vi "Begin.vi"(8 "error in":errorcluster) -> (0 "error out":errorcluster)   [LabVIEW 2020]
doc: "Called before other user functions, this VI is expected to open initial I/O refnums, load in file data, and do all program initialization. Notice that the <B>error out</B> terminal is simply used for data flow. Wiring it to other structures or subVIs ensures that this VI runs first."
uses:
  <vilib>/Rock Robotics/WPI/DriverStation/WPI_DriverStationRobotMode2.ctl
  <vilib>/Rock Robotics/WPI/Joystick/WPI_JoystickDeviceEnum.ctl
  <vilib>/Rock Robotics/WPI/SafetyOutput/WPI_SafetyOutputConfigMenu.ctl
  Robot Global Data.vi
  <vilib>/Rock Robotics/Network Tables/NT Write String Array.vi
  <vilib>/Rock Robotics/WPI/RobotDrive/WPI_RobotDriveOpen2MotorWithExistingMotors.vi
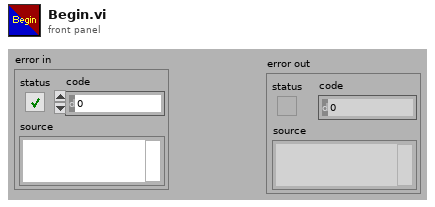
[diagram p1: front panel]
types:
  T1 = typedef "WPI_SafetyOutputConfigMenu.ctl" = enum16{"Enable", "Disable"}
  T2 = typedef "WPI_JoystickDeviceEnum.ctl" = enum16{"USB 0", "USB 1", "USB 2", "USB 3", "USB 4", "USB 5"}
  T3 = typedef "WPI_DriverStationRobotMode2.ctl" = enum16{"Autonomous Disabled", "Autonomous Enabled", "Teleop Disabled", "Teleop Enabled", "Disconnected", "Finish", "Test Disabled", "Test Enabled", "Emergency Stopped"}
  T4 = typedef "WPI_MotorControlDeviceRef.ctl" = cluster{"DeviceStatus":errorcluster, "Type":T5, "PWM":cluster{"PWM Channel":T6, "DeadBand":T7}, "CAN":cluster{"Device Number":u8, "SetOutput VI Ref":variant, "GetOutput VI Ref":variant, "Enable VI Ref":variant, "Disable VI Ref":variant, "Data":variant}, "Invert":bool, "DIO PWM":cluster{"PWM \"Enable\" Channel":T6, "DIOChannel":T8, "PWM Rate":dbl}}
  T5 = typedef "WPI_MotorControlType.ctl" = enum16{"PWM", "CAN", "DIO PWM"}
  T6 = typedef "FPGA_DIOPWMChannel.ctl" = enum8{"PWM 0", "PWM 1", "PWM 2", "PWM 3", "PWM 4", "PWM 5", "PWM 6", "PWM 7", "PWM 8", "PWM 9", "PWM MXP 0", "PWM MXP 1", "PWM MXP 2", "PWM MXP 3", "PWM MXP 4", "PWM MXP 5", "PWM MXP 6", "PWM MXP 7", "PWM MXP 8", "PWM MXP 9", "Invalid"}
  T7 = typedef "WPI_PWMDeadband.ctl" = cluster{"Name":string, "maxPositivePwm":i32, "minPositivePwm":i32, "centerPwm":i32, "maxNegativePwm":i32, "minNegativePwm":i32, "angularRange":u16}
  T8 = typedef "FPGA_DIOChannel.ctl" = enum8{"DIO 0", "DIO 1", "DIO 2", "DIO 3", "DIO 4", "DIO 5", "DIO 6", "DIO 7", "DIO 8", "DIO 9", "DIO MXP 0", "DIO MXP 1", "DIO MXP 2", "DIO MXP 3", "DIO MXP 4", "DIO MXP 5", "DIO MXP 6", "DIO MXP 7", "DIO MXP 8", "DIO MXP 9", "DIO MXP 10", "DIO MXP 11", "DIO MXP 12", "DIO MXP 13", "DIO MXP 14", "DIO MXP 15", "SPI Port CS1", "SPI Port CS2", "SPI Port CS3", "SPI Port MISO", "SPI Port MOSI", "Invalid"}
  T9 = typedef "WPI_JoystickDevRef.ctl" = cluster{"Device":T2}
  T10 = typedef "WPI_RobotDriveDevRef.ctl" = cluster{"DevStatus":errorcluster, "Motors[]":T4[], "Square Inputs":bool, "Max Output":dbl}
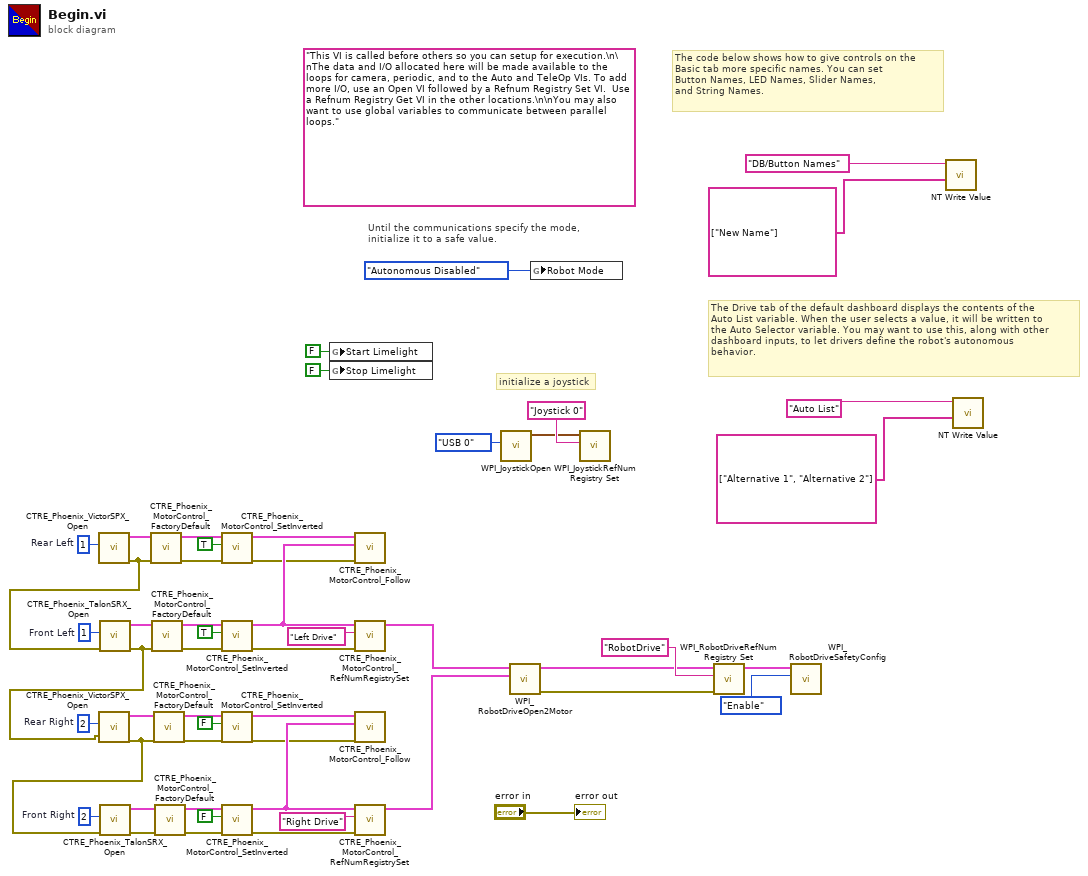
[diagram p0: block diagram]
diagram:
  w35 = u8 2  # Front Right
  w34 = u8 2  # Rear Right
  w33 = u8 1  # Front Left
  w32 = u8 1  # Rear Left
  (unwired) "This VI is called before others so you can setup for execution.\n\nThe data and I/O allocated here will be made available to the loops for camera, periodic, and to the Auto and TeleOp VIs. To add more I/O, use an Open VI followed by a Refnum Registry Set VI.  Use a Refnum Registry Get VI in the other locations.\n\nYou may also want to use global variables to communicate between parallel loops."
  # "The Drive tab of the default dashboard displays the contents of the\nAuto List variable. When the user selects a value, it will be written to\nthe Auto Selector variable. You may want to use this, along with other\ndashboard inputs, to let drivers define the robot's autonomous\nbehavior."
  # "The code below shows how to give controls on the\nBasic tab more specific names. You can set\nButton Names, LED Names, Slider Names,\nand String Names."
  # "initialize a joystick"
  # "Until the communications specify the mode,\ninitialize it to a safe value."
  n1 = call <vilib>:"CTRE_Phoenix_VictorSPX_Open.vi"("Device Number"=w32) -> ("error out"=w38:errorcluster, "PhoenixMotorControlDevRef"=w5:T4)  [unwired: 9 in]
  n2 = call <vilib>:"CTRE_Phoenix_TalonSRX_Open.vi"("error in"=w38, "Device Number"=w33) -> ("error out"=w39:errorcluster, "PhoenixMotorControlDevRef"=w11:T4)  [unwired: 8 in]
  n3 = call <vilib>:"CTRE_Phoenix_VictorSPX_Open.vi"("error in"=w39, "Device Number"=w34) -> ("error out"=w40:errorcluster, "PhoenixMotorControlDevRef"=w6:T4)  [unwired: 8 in]
  n4 = call <vilib>:"CTRE_Phoenix_TalonSRX_Open.vi"("error in"=w40, "Device Number"=w35) -> ("error out"=w12:errorcluster, "PhoenixMotorControlDevRef"=w13:T4)  [unwired: 8 in]
  n5 = call <vilib>:"CTRE_Phoenix_MotorControl_FactoryDefault.vi"("error in"=w38, "PhoenixMotorControlDevRef"=w5) -> ("error out"=w9:errorcluster, "PhoenixMotorControlDevRef"=w10:T4)  [unwired: 8 in]
  n6 = call <vilib>:"CTRE_Phoenix_MotorControl_FactoryDefault.vi"("error in"=w39, "PhoenixMotorControlDevRef"=w11) -> ("error out"=w16:errorcluster, "PhoenixMotorControlDevRef"=w17:T4)  [unwired: 8 in]
  n7 = call <vilib>:"CTRE_Phoenix_MotorControl_FactoryDefault.vi"("error in"=w40, "PhoenixMotorControlDevRef"=w6) -> ("error out"=w7:errorcluster, "PhoenixMotorControlDevRef"=w8:T4)  [unwired: 8 in]
  n8 = call <vilib>:"CTRE_Phoenix_MotorControl_FactoryDefault.vi"("error in"=w12, "PhoenixMotorControlDevRef"=w13) -> ("error out"=w14:errorcluster, "PhoenixMotorControlDevRef"=w15:T4)  [unwired: 8 in]
  n9 = call <vilib>:"CTRE_Phoenix_MotorControl_SetInverted.vi"("error in (no error)"=w9, "Invert?"=TRUE, "PhoenixMotorControlDevRef"=w10) -> ("error out"=w20:errorcluster, "PhoenixMotorControlDevRef"=w21:T4)  [unwired: 7 in]
  n10 = call <vilib>:"CTRE_Phoenix_MotorControl_SetInverted.vi"("error in (no error)"=w16, "Invert?"=TRUE, "PhoenixMotorControlDevRef"=w17) -> ("error out"=w18:errorcluster, "PhoenixMotorControlDevRef"=w28:T4)  [unwired: 7 in]
  n11 = call <vilib>:"CTRE_Phoenix_MotorControl_SetInverted.vi"("error in (no error)"=w7, "Invert?"=FALSE, "PhoenixMotorControlDevRef"=w8) -> ("error out"=w22:errorcluster, "PhoenixMotorControlDevRef"=w23:T4)  [unwired: 7 in]
  n12 = call <vilib>:"CTRE_Phoenix_MotorControl_SetInverted.vi"("error in (no error)"=w14, "Invert?"=FALSE, "PhoenixMotorControlDevRef"=w15) -> ("error out"=w19:errorcluster, "PhoenixMotorControlDevRef"=w29:T4)  [unwired: 7 in]
  n13 = global write "Robot Global Data.vi" "Start Limelight"(FALSE ("Start Limelight")) -> ()
  n14 = global write "Robot Global Data.vi" "Stop Limelight"(FALSE ("Stop Limelight")) -> ()
  n15 = call <vilib>:"CTRE_Phoenix_MotorControl_Follow.vi"("error in (no error)"=w20, "Master Controller to Follow"=w28, "PhoenixMotorControlDevRef"=w21) -> ()  [unwired: 7 in, 2 out]
  n16 = call <vilib>:"CTRE_Phoenix_MotorControl_RefNumRegistrySet.vi"("error in (no error)"=w18, "refnum name"="Left Drive", "PhoenixMotorControlDevRef"=w28) -> ("PhoenixMotorControlDevRef"=w36:T4)  [unwired: 7 in, 1 out]
  n17 = call <vilib>:"CTRE_Phoenix_MotorControl_Follow.vi"("error in (no error)"=w22, "Master Controller to Follow"=w29, "PhoenixMotorControlDevRef"=w23) -> ()  [unwired: 7 in, 2 out]
  n18 = call <vilib>:"CTRE_Phoenix_MotorControl_RefNumRegistrySet.vi"("error in (no error)"=w19, "refnum name"="Right Drive", "PhoenixMotorControlDevRef"=w29) -> ("PhoenixMotorControlDevRef"=w37:T4)  [unwired: 7 in, 1 out]
  n19 = call <vilib>:"WPI_JoystickOpen.vi"("JoystickDevice"=WPI_JoystickDeviceEnum."USB 0") -> ("JoystickDevRef"=w50:T9)  [unwired: 10 in]
  n20 = call-poly <vilib>:"WPI_RobotDriveOpen2Motor.vi"("Right Motor Dev Ref"=w37, "Left Motor Dev Ref"=w36) -> ("error out"=w3:errorcluster, "RobotDriveDevRef"=w4:T10)  [unwired: 3 in, 5 out]
  n21 = global write "Robot Global Data.vi" "Robot Mode"(WPI_DriverStationRobotMode2."Autonomous Disabled" ("Robot Mode")) -> ()
  n22 = call <vilib>:"WPI_JoystickRefNum Registry Set.vi"("refnum name"="Joystick 0", "JoystickDevRef"=w50) -> ()  [unwired: 8 in, 2 out]
  n23 = call <vilib>:"WPI_RobotDriveRefNum Registry Set.vi"("error in (no error)"=w3, "refnum name"="RobotDrive", "RobotDriveDevRef"=w4) -> ("RobotDriveDevRef"=w43:T10)  [unwired: 1 in, 7 out]
  n24 = call <vilib>:"WPI_RobotDriveSafetyConfig.vi"("mode"=WPI_SafetyOutputConfigMenu."Enable", "RobotDriveDevRef"=w43) -> ()  [unwired: 8 in, 2 out]
  n25 = call-poly <vilib>:"NT Write Value.vi"("String Array"=string[] ["New Name"], "Name"="DB/Button Names") -> ()  [unwired: 9 in, 1 out]
  n26 = call-poly <vilib>:"NT Write Value.vi"("String Array"=string[] ["Alternative 1", "Alternative 2"], "Name"="Auto List") -> ()  [unwired: 9 in, 1 out]
  "error out" <- "error in"
